vi "Pre Launch Init.vi"(11 "DATABASE in":refnum<class "DATABASE.lvclass">) -> (0 "error out":errorcluster, 3 "DATABASE out":refnum<class "DATABASE.lvclass">)   [LabVIEW 2019, in "DATABASE.lvlib" / "DATABASE.lvclass"]
doc: "(<B>Filename</B>: Actor Framework.lvlib:Actor.lvclass:Pre Launch Init.vi)\n\nDefines behavior that occurs after the Launch Nested Actor method is invoked but before the actor's Actor Core method begins running.\n\nBy default, this method does nothing. A descendant class may override it to define behavior."
uses:
  DATABASE.lvclass
  DATABASE.lvclass/DATABASE.ctl
  <vilib>/ActorFramework/Actor/Actor.lvclass
panel:
  in  "EXIT":bool
  in  "BASE_DE_DATOS":string
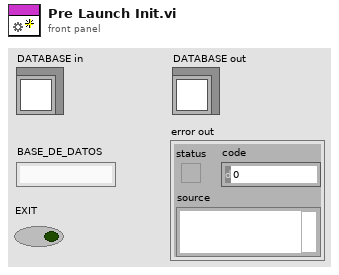
[diagram p1: front panel]
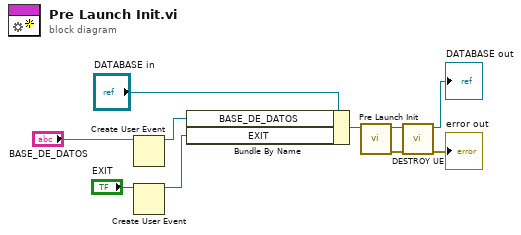
[diagram p0: block diagram]
diagram:
  n1 = Create User Event(user event datatype="BASE_DE_DATOS") -> (user event=w6:refnum<user-event>)  [unwired: 1 in, 1 out]
  n2 = Create User Event(user event datatype="EXIT") -> (user event=w5:refnum<user-event>)  [unwired: 1 in, 1 out]
  n3 = Bundle By Name(cluster="DATABASE in", "BASE_DE_DATOS"=w6, "EXIT"=w5) -> (w7:refnum<class "DATABASE.lvclass">)
  n4 = call-parent "Pre Launch Init.vi"("Actor in"=w7) -> ("error out"=w4:errorcluster, "Actor out"=w1:refnum<class "DATABASE.lvclass">)  [unwired: 9 in]
  n5 = call "DESTROY UE.vi"("error in (no error)"=w4, "DATABASE in"=w1) -> ("error out"=→"error out":errorcluster, "DATABASE out"=→"DATABASE out":refnum<class "DATABASE.lvclass">)  [unwired: 8 in]
